vi "mVreader.vi"() -> (3 "Numeric":dbl)   [LabVIEW 2012]
panel:
  out "error out":errorcluster
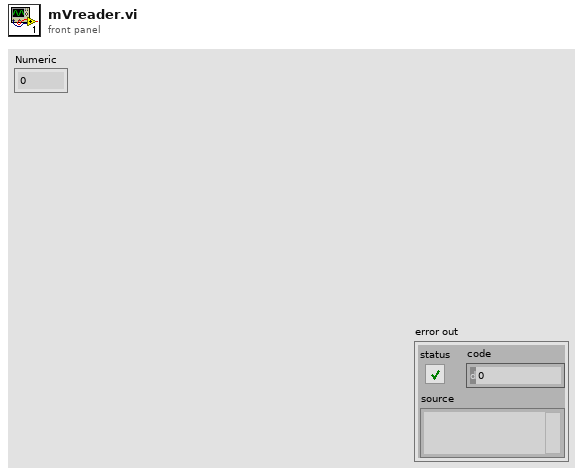
[diagram p1: front panel]
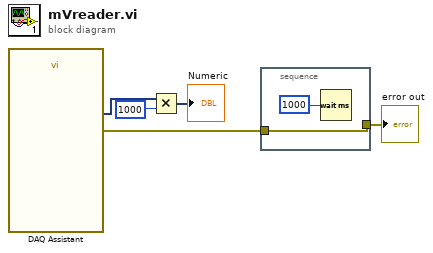
[diagram p0: block diagram]
diagram:
  n1 = call "DAQ Assistant"() -> ("data"=w4:dynamicdata, "error out"=w1:errorcluster)  [unwired: 17 in, 1 out]
  n2 = Multiply(x=w4, y=1000) -> (x*y=→"Numeric":dynamicdata)
  n3 = stacked-sequence {
    tunnel: [w6] -> w5
    tunnel: w1 -> [w6]
    frame #0 {
      n4 = Wait (ms)(milliseconds to wait=u32 1000) -> ()  [unwired: 1 out]
    }
  }
  "error out" <- w5
